vi "direction.vi"(7 "LabVIEW Web Service Request":refnum<class "Web Request.lvclass">, 11 "name":string) -> (3 "value":string)   [LabVIEW 2015]
uses:
  <vilib>/wsapi/Web Request.lvclass
panel:
  # "Use the Web Service Request input terminal to call the VIs on the Web Services palette. Do not remove it from the connector pane unless you don't need access to the palette."
  # "Each additional control wired to the connector pane will be available as an input in the URL. To include an indicator in terminal-mode output (the default setting), it must also be wired to the connector pane."
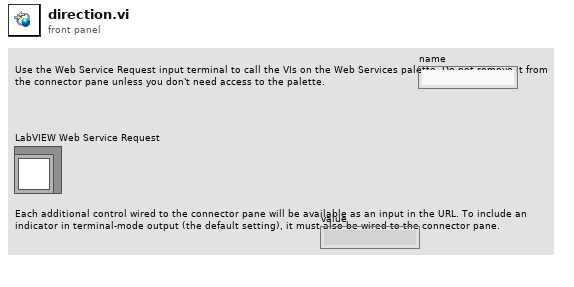
[diagram p1: front panel]
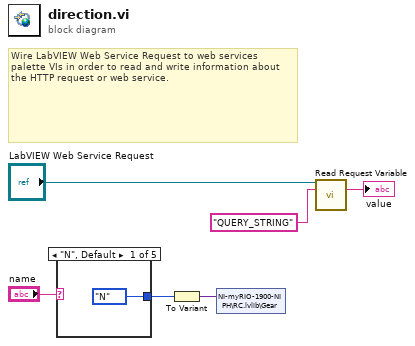
[diagram p0: block diagram]
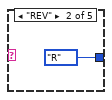
[diagram p2: hidden frame]
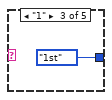
[diagram p3: hidden frame]
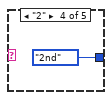
[diagram p4: hidden frame]
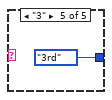
[diagram p5: hidden frame]
diagram:
  # "Wire LabVIEW Web Service Request to web services palette VIs in order to read and write information about the HTTP request or web service."
  n1 = case shown="\"N\", Default" "name" {
    tunnel: [enum16{"3rd", "2nd", "1st", "N", "R"}."N" ("Enum") enum16{"3rd", "2nd", "1st", "N", "R"}."R" ("Enum") enum16{"3rd", "2nd", "1st", "N", "R"}."1st" ("Enum") enum16{"3rd", "2nd", "1st", "N", "R"}."2nd" ("Enum") enum16{"3rd", "2nd", "1st", "N", "R"}."3rd" ("Enum")] -> w1
    frame "N", Default {
    }
    frame "REV" {
    }
    frame "1" {
    }
    frame "2" {
    }
    frame "3" {
    }
  }
  n2 = To Variant(anything=w1) -> (Variant=w2:variant)
  n3 = shared-variable "NI-myRIO-1900-NIPH\\RC.lvlib\\Gear"(w2) -> ()  [unwired: 1 in, 1 out]
  n4 = call <vilib>:"Read Request Variable.vi"("LabVIEW Web Service Request"="LabVIEW Web Service Request", "variable name"="QUERY_STRING") -> ("value"=→"value":string)  [unwired: 11 in, 2 out]
